vi "Multi_Stage_Resample.vi"(5 "X Resolution":i32, 7 "Y Resolution":i32, 8 "error in (no error)":errorcluster, 9 "Interpolation Type":u32(ring)=1 items=["Zero Order", "Bi-Linear", "Quadratic", "Cubic Spline"], 10 "Img in":T1, 11 "Dest":T1) -> (0 "error out":errorcluster, 3 "Img out":T1)   [LabVIEW 2024]
uses:
  <vilib>/vision/Image Controls.llb/IMAQ Image.ctl
  <vilib>/vision/NI_Vision_Development_Module.lvlib
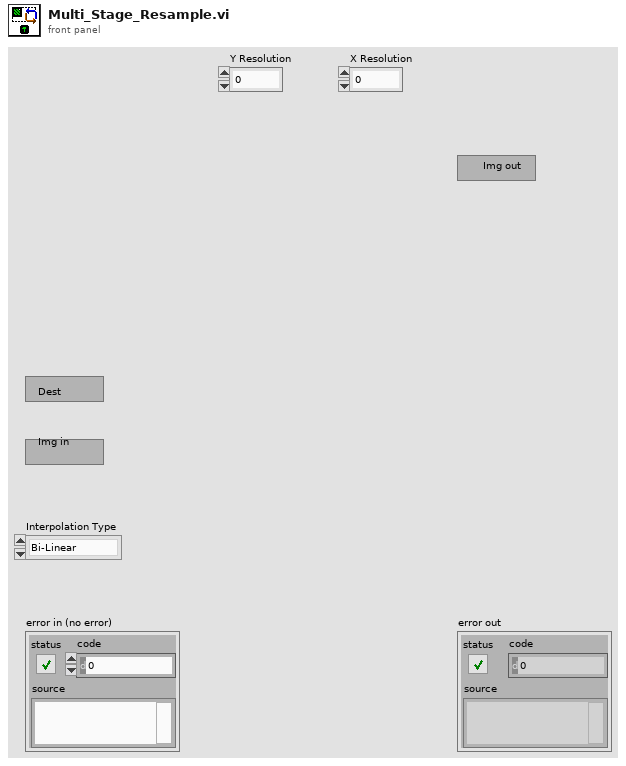
[diagram p1: front panel]
types:
  T1 = typedef "IMAQ Image.ctl" = refnum<image>
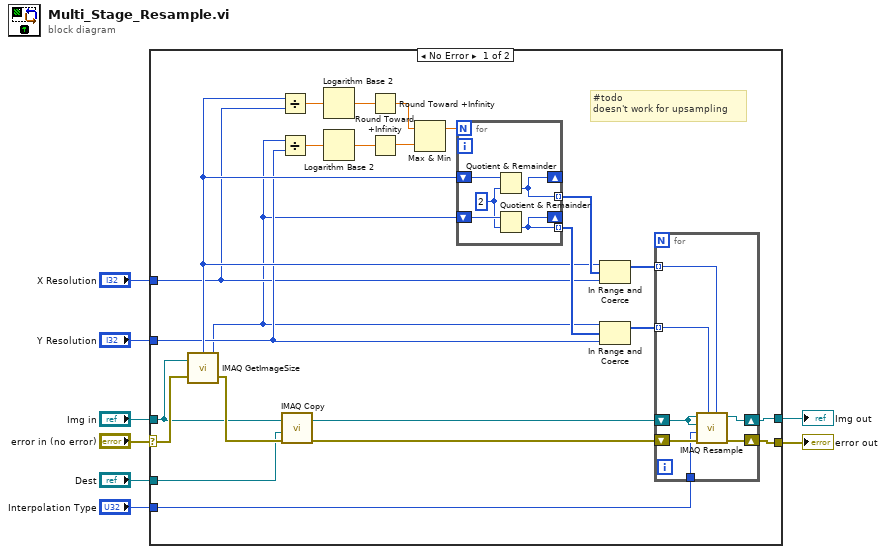
[diagram p0: block diagram]
diagram:
  n1 = case shown="No Error" "error in (no error)" {
    selector: "error in (no error)" -> [w31 w45]
    tunnel: [w27 w45] -> w7
    tunnel: [w26 w46] -> w6
    tunnel: "Img in" -> [w14 w46]
    tunnel: "Dest" -> [w13 _]
    tunnel: "Interpolation Type" -> [w12 _]
    tunnel: "Y Resolution" -> [w11 _]
    tunnel: "X Resolution" -> [w10 _]
    frame No Error {
      # "#todo\ndoesn't work for upsampling"
      n2 = call "IMAQ GetImageSize"("Image"=w14, "error in (no error)"=w31) -> ("Y Resolution"=w9:i32, "X Resolution"=w15:i32, "error out"=w32:errorcluster)  [unwired: 2 in]
      n3 = Divide(x=w15, y=w10) -> (x/y=w24:dbl)
      n4 = Divide(x=w9, y=w11) -> (x/y=w22:dbl)
      n5 = call "IMAQ Copy"("error in (no error)"=w32, "Image Dst"=w13, "Image Src"=w14) -> ("error out"=w29:errorcluster, "Image Dst Out"=w28:T1)  [unwired: 3 in]
      n6 = Logarithm Base 2(1:w24) -> (0:w23:dbl)
      n7 = Logarithm Base 2(1:w22) -> (0:w25:dbl)
      n8 = Round Toward +Infinity(x=w23) -> (ceil(x): smallest int >= x=w21:dbl)
      n9 = Round Toward +Infinity(x=w25) -> (ceil(x): smallest int >= x=w30:dbl)
      n10 = Max & Min(x=w21, y=w30) -> (max(x,y)=w20:dbl)  [unwired: 1 out]
      n11 = for {
        N: w20 -> [_]
        tunnel: [w42] -> w19 mode=indexing
        tunnel: [w41] -> w18 mode=indexing
        shift-right: [w41] -> _
        shift-left: w15 -> [w44]
        shift-right: [w42] -> _
        shift-left: w9 -> [w43]
        w40 = 2 ("y")
        n12 = Quotient & Remainder(x=w44, y=w40) -> (floor(x/y)=w41:i32)  [unwired: 1 out]
        n13 = Quotient & Remainder(x=w43, y=w40) -> (floor(x/y)=w42:i32)  [unwired: 1 out]
      }
      n14 = In Range and Coerce(upper limit=w15, x=w18, lower limit=w10) -> (coerced(x)=w17:i32[])  [unwired: 1 out]
      n15 = In Range and Coerce(upper limit=w9, x=w19, lower limit=w11) -> (coerced(x)=w16:i32[])  [unwired: 1 out]
      n16 = for {
        shift-right: [w38] -> w27
        shift-left: w29 -> [w39]
        shift-right: [w37] -> w26
        shift-left: w28 -> [w34]
        tunnel: w16 -> [w36] mode=indexing
        tunnel: w17 -> [w35] mode=indexing
        tunnel: w12 -> [w33]
        n17 = call "IMAQ Resample"("X Resolution"=w35, "Y Resolution"=w36, "error in (no error)"=w39, "Interpolation Type"=w33, "Image Dst"=w34, "Image Src"=w34) -> ("error out"=w38:errorcluster, "Image Dst Out"=w37:T1)  [unwired: 4 in]
      }
    }
    frame Error {
    }
  }
  "error out" <- w7
  "Img out" <- w6
